vi "pre-bias.vi"(7 "error in (no error)":errorcluster, 9 "Check scan settings":T1 {"Logarithmic sweep" items=["False", "True"]; "Repeat scans" items=["True", "False"]; "No. of repeat scans" min=1.0 step=1.0; "Stabilisation mode" items=["V", "I"]; "Dual sweep" items=["True", "False"]; "Measurement delay (ms)" min=10.0}, 10 "VISA resource name in":refnum<visa-resource-name>) -> (0 "error out":errorcluster, 2 "Stabilisation data":dbl[][](array[numeric]), 3 "VISA resource name out":refnum<visa-resource-name>)   [LabVIEW 2016]
uses:
  TypeDefs/settings.ctl
  C:/Program Files (x86)/National Instruments/LabVIEW 2016/instr.lib/keithley_24xx/Keithley 24XX/Public/Data/Read (Single Point).vi
  C:/Program Files (x86)/National Instruments/LabVIEW 2016/instr.lib/keithley_24xx/Keithley 24XX/Keithley 24XX.lvlib
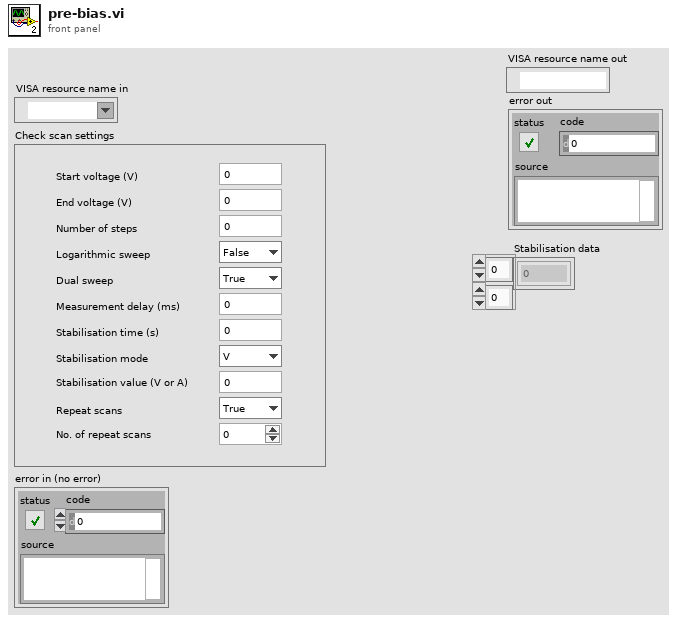
[diagram p1: front panel]
types:
  T1 = typedef "settings.ctl" = cluster{"Start voltage (V)":dbl, "End voltage (V)":dbl, "Number of steps":u32, "Measurement delay (ms)":dbl, "Dual sweep":u16, "Stabilisation time (s)":dbl, "Stabilisation mode":u16, "Stabilisation value (V or A) ":dbl, "No. of repeat scans":dbl, "Repeat scans":u16, "Logarithmic sweep":u16}
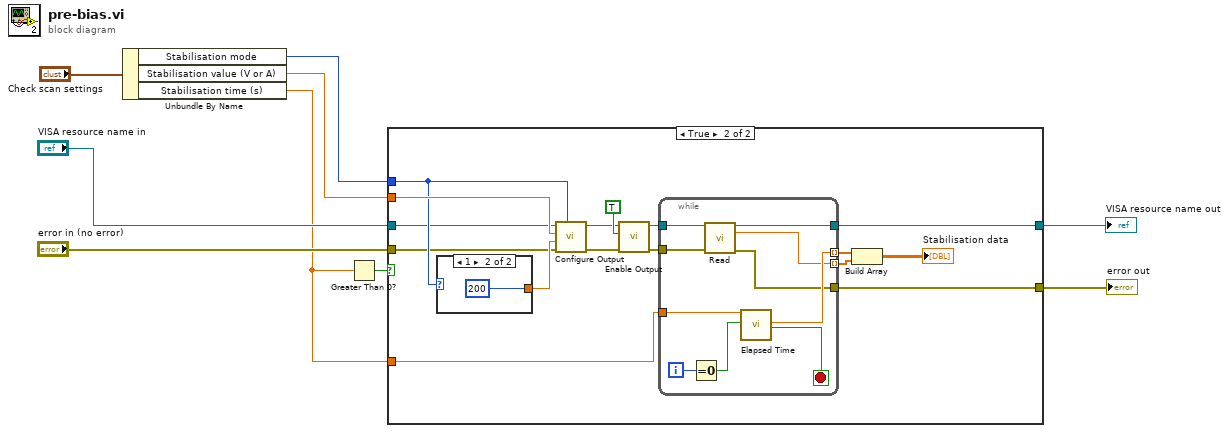
[diagram p0: block diagram]
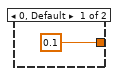
[diagram p3: hidden frame]
diagram:
  n1 = Unbundle By Name("Check scan settings") -> ("Stabilisation mode"=w8:u16, "Stabilisation value (V or A)"=w9:dbl, "Stabilisation time (s)"=w1:dbl)
  n2 = Greater Than 0?(x=w1) -> (x > 0?=w2:bool)
  n3 = case shown="True" w2 {
    tunnel: w1 -> [_ w25]
    tunnel: w9 -> [_ w24]
    tunnel: w8 -> [_ w23]
    tunnel: "error in (no error)" -> [w10 w22]
    tunnel: "VISA resource name in" -> [w11 w21]
    tunnel: [w11 w13] -> w4
    tunnel: [w10 w12] -> w3
    frame False {
    }
    frame True {
      n4 = case shown="1" w23 {
        tunnel: [0.1 200] -> w27
        frame 0, Default {
        }
        frame 1 {
        }
      }
      n5 = call "Configure Output.vi"("Source Mode  (0: Voltage)"=w23, "error in (no error)"=w22, "Compliance  Level (0.1)"=w27, "Output Level (0)"=w24, "VISA resource name"=w21) -> ("error out"=w14:errorcluster, "VISA resource name out"=w15:refnum<visa-resource-name>)  [unwired: 5 in]
      n6 = call "Enable Output.vi"("error in (no error)"=w14, "Enable Output (T: Enable)"=TRUE ("Output (Off)"), "VISA resource name"=w15) -> ("error out"=w18:errorcluster, "VISA resource name out"=w17:refnum<visa-resource-name>)  [unwired: 7 in]
      n7 = while {
        tunnel: w17 -> [w39]
        tunnel: w18 -> [w38]
        tunnel: [w37] -> w13
        tunnel: [w35] -> w19 mode=indexing
        tunnel: [w34] -> w20 mode=indexing
        tunnel: w25 -> [w31]
        tunnel: [w30] -> w12
        i -> [w33]
        stop <- w36 stop-if-true
        n8 = Equal To 0?(x=w33) -> (x = 0?=w32:bool)
        n9 = call-poly "Read.vi"("VISA resource name"=w39, "error in (no error)"=w38) -> ("VISA resource name out"=w37:refnum<visa-resource-name>, "Current"=w34:sgl, "error out"=w30:errorcluster)  [unwired: 7 in, 4 out]
        n10 = call "Elapsed Time"("Time Target (s)"=w31, "Reset"=w32) -> ("Elapsed Time (s)"=w35:dbl, "Time has Elapsed"=w36:bool)  [unwired: 10 in, 6 out]
      }
      n11 = Build Array(w19, w20) -> (→"Stabilisation data":dbl[][])
    }
  }
  "VISA resource name out" <- w4
  "error out" <- w3
